vi "Copy Boolean Caption to BooleanText.vi"(6 "Variant in":variant, 7 "Shift Pressed?":bool, 8 "error in (no error)":errorcluster, 10 "QD Combo Box Ref":refnum<vi>, 11 "QD Launch VI Ref":refnum<vi>) -> (0 "error out":errorcluster, 4 "Variant out":variant)   [LabVIEW 2014, in "NEVSTOP_QuickDrop.lvlib"]
doc: "Write a 1-2 sentence description of the functionality of your plugin here. Replace the \"$\" below with the character you wish to assign as the default shortcut for this plugin. Do not add any text after the 'Default Shortcut' line below.\n\nDefault Shortcut - [$]"
uses:
  NEVSTOP_QuickDrop.lvlib
panel:
  in  "Undo Name":string="Quick Drop Keyboard Shortcut"
  # "Do not change the connector pane of this VI.\n\nSee the block diagram for directions on how to use this template."
  # "Specify the name of the Undo transaction"
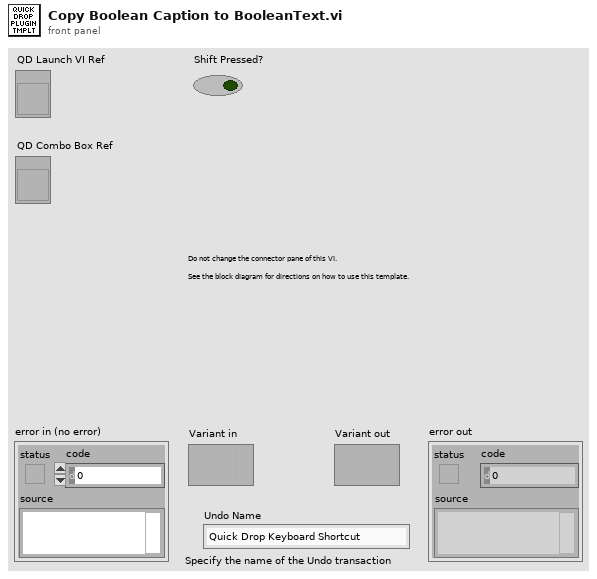
[diagram p1: front panel]
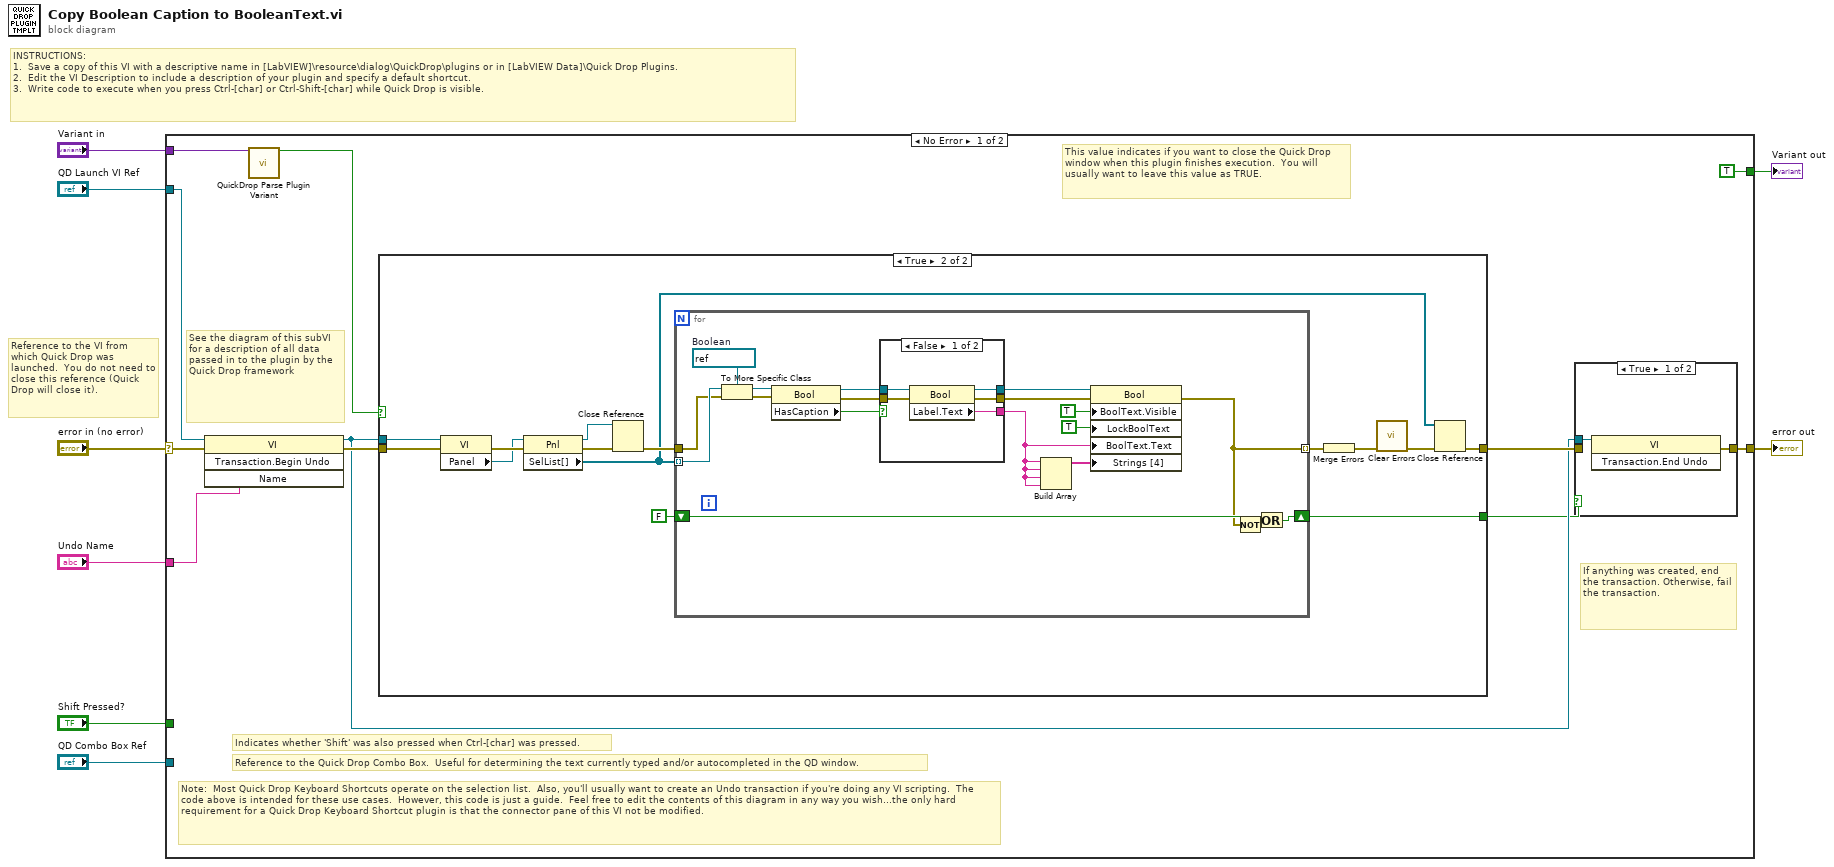
[diagram p0: block diagram]
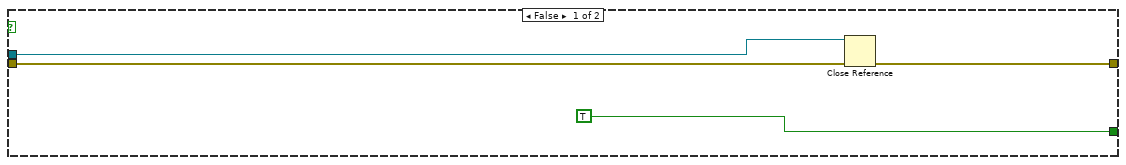
[diagram p2: hidden frame]
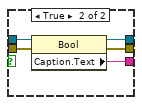
[diagram p3: hidden frame]
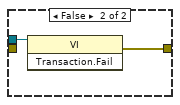
[diagram p4: hidden frame]
diagram:
  # "Reference to the VI from which Quick Drop was launched.  You do not need to close this reference (Quick Drop will close it)."
  # "INSTRUCTIONS:\n1.  Save a copy of this VI with a descriptive name in [LabVIEW]\\resource\\dialog\\QuickDrop\\plugins or in [LabVIEW Data]\\Quick Drop Plugins.\n2.  Edit the VI Description to include a description of your plugin and specify a default shortcut. \n3.  Write code to execute when you press Ctrl-[char] or Ctrl-Shift-[char] while Quick Drop is visible."
  n1 = case shown="No Error" "error in (no error)" {
    selector: "error in (no error)" -> [w18 w70]
    tunnel: [w12 w70] -> w7
    tunnel: "QD Launch VI Ref" -> [w17 _]
    tunnel: "Shift Pressed?" -> [_ _]
    tunnel: "QD Combo Box Ref" -> [_ _]
    tunnel: "Variant in" -> [w19 _]
    tunnel: "Undo Name" -> [w16 _]
    tunnel: [TRUE _] -> w1
    frame No Error {
      # "Note:  Most Quick Drop Keyboard Shortcuts operate on the selection list.  Also, you'll usually want to create an Undo transaction if you're doing any VI scripting.  The code above is intended for these use cases.  However, this code is just a guide.  Feel free to edit the contents of this diagram in any way you wish...the only hard requirement for a Quick Drop Keyboard Shortcut plugin is that the connector pane of this VI not be modified."
      # "If anything was created, end the transaction. Otherwise, fail the transaction."
      # "This value indicates if you want to close the Quick Drop window when this plugin finishes execution.  You will usually want to leave this value as TRUE."
      # "See the diagram of this subVI for a description of all data passed in to the plugin by the Quick Drop framework"
      # "Reference to the Quick Drop Combo Box.  Useful for determining the text currently typed and/or autocompleted in the QD window."
      # "Indicates whether 'Shift' was also pressed when Ctrl-[char] was pressed."
      n2 = invoke class="VI" method="Transaction.Begin Undo"(reference=w17, error in=w18, "Name"=w16) -> (reference out=w10:refnum<vi>, error out=w13:errorcluster)  [unwired: 1 in, 2 out]
      n3 = call <vilib>:"QuickDrop Parse Plugin Variant.vi"("QDKS Variant in"=w19) -> ("QD Launch VI Panel?"=w14:bool)  [unwired: 12 in, 2 out]
      n4 = case shown="True" w14 {
        tunnel: w13 -> [w22 w37]
        tunnel: [w21 w27] -> w11
        tunnel: w10 -> [w20 w35]
        tunnel: [TRUE w33] -> w9
        frame False {
          n5 = Close Reference(reference=w20, error in (no error)=w22) -> (error out=w21:errorcluster)
        }
        frame True {
          n6 = property class="VI"(reference=w35, error in=w37) -> (error out=w32:errorcluster, "Panel"=w31:refnum<vi>)  [unwired: 1 out]
          n7 = property class="Pnl"(reference=w31, error in=w32) -> (reference out=w29:refnum<vi>, error out=w30:errorcluster, "SelList[]"=w26:refnum<vi>[])
          n8 = Close Reference(reference=w29, error in (no error)=w30) -> (error out=w36:errorcluster)
          n9 = for {
            shift-right: [w54] -> w33
            shift-left: FALSE -> [w55]
            tunnel: w26 -> [w53] mode=indexing
            tunnel: w36 -> [w51]
            tunnel: [w41] -> w28 mode=indexing
            w52 = refnum<vi> refnum  # Boolean
            n10 = To More Specific Class(target class=w52, reference=w53, error in=w51) -> (specific class reference=w50:refnum<vi>, error out=w49:errorcluster)
            n11 = property class="Bool"(reference=w50, error in=w49) -> (reference out=w47:refnum<vi>, error out=w48:errorcluster, "HasCaption"=w46:bool)
            n12 = case shown="False" w46 {
              tunnel: w48 -> [w59 w65]
              tunnel: w47 -> [w60 w64]
              tunnel: [w57 w63] -> w45
              tunnel: [w58 w62] -> w44
              tunnel: [w56 w61] -> w38
              frame False {
                n13 = property class="Bool"(reference=w60, error in=w59) -> (reference out=w57:refnum<vi>, error out=w58:errorcluster, "Label.Text"=w56:string)
              }
              frame True {
                n14 = property class="Bool"(reference=w64, error in=w65) -> (reference out=w63:refnum<vi>, error out=w62:errorcluster, "Caption.Text"=w61:string)
              }
            }
            n15 = Build Array(w38, w38, w38, w38) -> (w39:string[])
            n16 = property class="Bool"(reference=w45, error in=w44, "BoolText.Visible"=TRUE ("Boolean Text.Visible"), "LockBoolText"=TRUE ("Lock Boolean Text In Center"), "BoolText.Text"=w38, "Strings [4]"=w39) -> (error out=w41:errorcluster)  [unwired: 1 out]
            n17 = Not(x=w41) -> (.not. x?=w40:bool)
            n18 = Or(x=w55, y=w40) -> (x .or. y?=w54:bool)
          }
          n19 = Merge Errors(w28) -> (w25:errorcluster)
          n20 = call <vilib>:"Clear Errors.vi"("error in (no error)"=w25) -> ("error out"=w24:errorcluster)  [unwired: 5 in, 1 out]
          n21 = Close Reference(reference=w26, error in (no error)=w24) -> (error out=w27:errorcluster)
        }
      }
      n22 = case shown="True" w9 {
        tunnel: w10 -> [w66 w68]
        tunnel: [w67 w69] -> w12
        tunnel: w11 -> [_ _]
        frame True {
          n23 = invoke class="VI" method="Transaction.End Undo"(reference=w66) -> (error out=w67:errorcluster)  [unwired: 2 in, 2 out]
        }
        frame False {
          n24 = invoke class="VI" method="Transaction.Fail"(reference=w68) -> (error out=w69:errorcluster)  [unwired: 2 in, 2 out]
        }
      }
    }
    frame Error {
    }
  }
  "error out" <- w7
  "Variant out" <- w1
